vi "IndexIncrement (SubVI).vi"(2 "array type (2D Dbl)":dbl[](array[numeric]), 3 "Index":dbl) -> (0 "Index+1":dbl, 1 "Out":dbl)   [LabVIEW 2013]
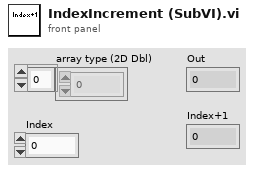
[diagram p1: front panel]
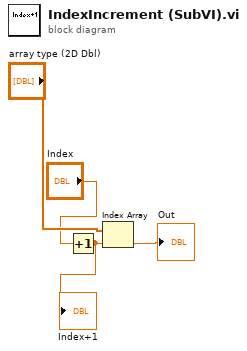
[diagram p0: block diagram]
diagram:
  n1 = Increment(x="Index") -> (x+1=w1:dbl)
  "Index+1" <- w1
  n2 = Index Array(array="array type (2D Dbl)", index=w1) -> (element=→"Out":dbl)
